vi "Publish User List.vi"(8 "error in (no error)":errorcluster, 11 "LV Chat Server in":refnum<class "LV Chat Server.lvclass">) -> (0 "error out":errorcluster, 3 "LV Chat Server out":refnum<class "LV Chat Server.lvclass">)   [LabVIEW 2020, in "LV Chat Server.lvclass"]
uses:
  LV Chat Server.lvclass
  Data Types/Message ID.ctl
  LV Chat Server.lvclass/LV Chat Server.ctl
  f0ba566d-872e-4f25-9af0-524adfd6c013.vi
  7433a138-1183-4426-b237-c60b61f96981.vi
  7433a138-1183-4426-b237-c60b61f96981.vi/43e93f4b-eb60-4448-b7e4-56a49cc750fb.vi
  7433a138-1183-4426-b237-c60b61f96981.vi/43e93f4b-eb60-4448-b7e4-56a49cc750fb.vi/4b61994f-5270-44fc-a580-5e93e6c23fba.vi
  <vilib>/IlluminatedG/lv-stream/stream/Write Formatted Data.vi
  <vilib>/IlluminatedG/lv-msg-simple/Stream-Simple-Msg/Manager/Get Endpoints.vi
  <vilib>/IlluminatedG/lv-msg-simple/Stream-Simple-Msg/Endpoint/Get Stream.vi
  <vilib>/IlluminatedG/lv-stream/stream/Get Mode.vi
  <vilib>/IlluminatedG/lv-stream/stream/Prepared.vi
  <vilib>/Utility/error.llb/Error Cluster From Error Code.vi
  <vilib>/IlluminatedG/lv-stream/stream/Dispatch Sniffer Data.vi
  <vilib>/IlluminatedG/lv-stream/stream/Stream.lvclass
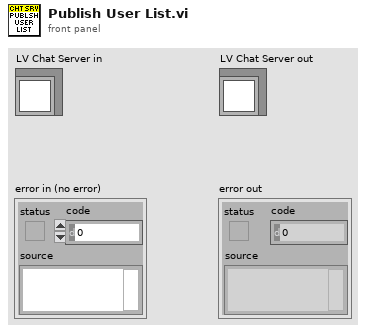
[diagram p1: front panel]
types:
  T1 = typedef "Message ID.ctl" = enum16{"UserInfo", "UserList", "Message", "Disconnect"}
  T2 = typedef "LV Chat Server.lvclass/Ref Data.ctl" = cluster{"Endpoint Map":map{string, T3}, "User Map":map{string, string}}
  T3 = typedef "LV Chat Server.lvclass/User.ctl" = cluster{"Name":string, "IP":string, "Connected At":dbl, "Endpoint":refnum<class "Endpoint.lvclass">}
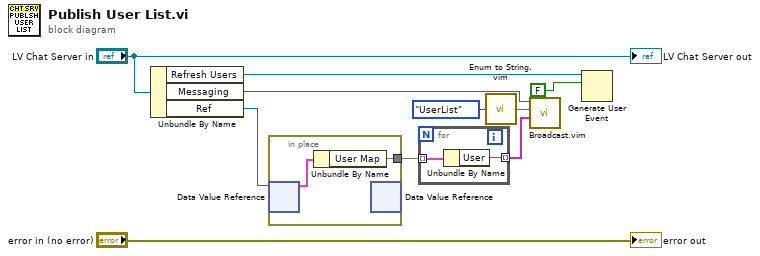
[diagram p0: block diagram]
diagram:
  n1 = Unbundle By Name("LV Chat Server in") -> ("Refresh Users"=w2:refnum<user-event>, "Messaging"=w8:refnum<class "Manager.lvclass">, "Ref"=w7:refnum<data-value>)
  n2 = in-place {
    in-place-border: [w11] -> w6
    n3 = in-place-dvr #1(w7) -> (w12:T2)  [unwired: 1 out]
    n4 = Unbundle By Name(w12) -> ("User Map"=w11:map{string, string})
    n5 = in-place-dvr #1() -> ()  [unwired: 1 in, 2 out]
  }
  n6 = for {
    tunnel: w6 -> [w14] mode=indexing
    tunnel: [w13] -> w5 mode=indexing
    n7 = Unbundle By Name(w14) -> ("User"=w13:string)
  }
  n8 = call "Enum to String.vim"("Enum"=Message_ID."UserList" ("Message ID")) -> ("Enum String"=w3:string)
  n9 = call "Broadcast.vim"("Data"=w5, "ID"=w3, "Manager in"=w8) -> ()  [unwired: 7 in, 2 out]
  n10 = Generate User Event(user event=w2, event data cluster=FALSE ("event data")) -> ()  [unwired: 2 in, 2 out]
  "error out" <- "error in (no error)"
  "LV Chat Server out" <- "LV Chat Server in"
